vi "Eval y=f(x) Prep.vi"(0 "formula":string, 1 "epsilon":dbl format="%.2f") -> (2 "error (formula)":bool, 3 "error (general)":bool, 4 "error (epsilon)":bool, 5 "List of variables":i32[](array[numeric]))   [LabVIEW 2010, in "NI_Gmath.lvlib"]
uses:
  NI_Gmath.lvlib
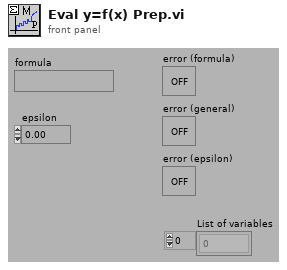
[diagram p1: front panel]
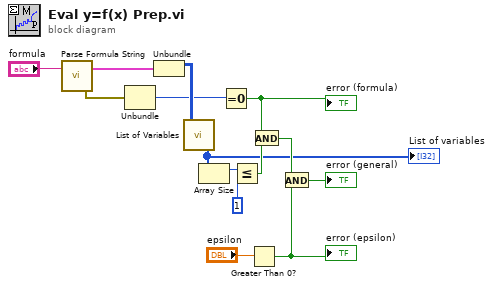
[diagram p0: block diagram]
diagram:
  n1 = call "Parse Formula String.vi"("formula"="formula") -> ("error out"=w4:errorcluster, "Parsed Formula"=w12:cluster{"Table":i32[][], "Y Values":dbl[]})  [unwired: 1 in]
  n2 = Unbundle(w4) -> ("code"=w5:i32)  [unwired: 2 out]
  n3 = Unbundle(w12) -> ("Table"=w13:i32[][])  [unwired: 1 out]
  n4 = call "List of Variables.vi"("Table"=w13) -> ("List of variables"=w3:i32[])
  "List of variables" <- w3
  n5 = Array Size(array=w3) -> (size(s)=w1:i32)
  n6 = Equal To 0?(x=w5) -> (x = 0?=w7:bool)
  "error (formula)" <- w7
  n7 = Less Or Equal?(x=w1, y=1) -> (x <= y?=w6:bool)
  n8 = Greater Than 0?(x="epsilon") -> (x > 0?=w11:bool)
  "error (epsilon)" <- w11
  n9 = And(x=w7, y=w6) -> (x .and. y?=w9:bool)
  n10 = And(x=w9, y=w11) -> (x .and. y?=→"error (general)":bool)
